vi "Close.vi"(8 "error in (no error)":errorcluster, 11 "ChromaAcLoad in":refnum<class "ChromaAcLoad.lvclass">) -> (0 "error out":errorcluster, 3 "ChromaAcLoad out":refnum<class "ChromaAcLoad.lvclass">)   [LabVIEW 2018, in "AcPwrPlugins.lvlib" / "ChromaAcLoad.lvclass"]
doc: "This VI closes the reference to the instrument(s)."
uses:
  ChromaAcLoad.lvclass
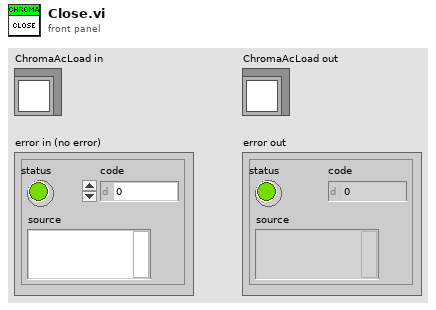
[diagram p1: front panel]
types:
  T1 = typedef "AcPwrPlugins.lvlib/ChromaAcLoad.lvclass/Device(s)Settings.ctl" = cluster{"Configuration Mode":T2, "Phases":cluster{"Handle":string, "Name":string, "Phase Select":i32, "Instrument Options":string, "id query (T)":bool, "reset device (T)":bool, "Load Short Circuited":bool, "Line Synchronization":bool, "Load Current (A/Arms)":dbl, "Load Voltage (V/Vrms)":dbl, "Load Power (W)":dbl, "Load Resistance (Ohms)":dbl, "Load Current Peak Limit (A)":dbl, "Load Current Limit (A/Arms)":dbl, "Load Power Limit (W)":dbl, "Synch Frequency (Hz)":dbl, "Priority":enum16{"CF Only", "PF Only", "Both (CF)", "Both (PF)"}, "Crest Factor":dbl, "Power Factor":dbl, "Slew Rate":cluster{"Rise Slew Rate (A/ms)":i32, "Fall Slew Rate (A/ms)":i32}, "LC/RLC Mode":cluster{"Capacitance (uF)":i32, "Inductance (uH)":i32, "Series Resistance (Ohm)":dbl, "Parallel Resistance (Ohm)":dbl}, "Timing":cluster{"TimingOn":enum16{""}, "Hours":u32, "Minutes":u32, "Seconds":dbl, "CutoffVoltage":dbl}, "Connected":bool}[], "MeasName":string}
  T2 = typedef "ConfigMode.ctl" = enum16{"Constant Voltage (DC)", "Constant Power (DC)", "Constant Power (AC)", "Constant Current (DC)", "Constant Current (AC)", "Constant Resistance (DC)", "Constant Resistance (AC)", "Rectified Mode (DC)", "Inrush (AC)", "RLC CP (AC)", "RLC (AC)"}
  T3 = typedef "AcPwrPlugins.lvlib/ChromaAcLoad.lvclass/Measurements.ctl" = cluster{"Handle":string, "Name":string, "Enabled":bool, "Measurement Value":dbl, "Hold Peak Current Measurement":bool, "btnMeasFetch":bool, "ProtectionStatusString":string, "Measurement Type":T4}[]
  T4 = typedef "AcPwrPlugins.lvlib/ChromaAcLoad.lvclass/MeasurementType.ctl" = enum16{"Voltage (Vrms or V)", "Current (Arms or A)", "Power (W)", "Peak Voltage (V)", "Peak Current (A)", "Peak Power (W)", "Frequency (Hz)", "Resistance (Ohms)", "Voltage Overshoot (V)", "Positive Peak Current (A)", "Voltage Undershoot (V)", "Negative Peak Current (A)", "Apparent Power (VA)", "Reacitive Power (VAR)", "Voltage THD", "Power Factor", "Current's Crest Factor"}
  T5 = cluster{"Handle":string, "Name":string, "Phase Select":i32, "Instrument Options":string, "id query (T)":bool, "reset device (T)":bool, "Load Short Circuited":bool, "Line Synchronization":bool, "Load Current (A/Arms)":dbl, "Load Voltage (V/Vrms)":dbl, "Load Power (W)":dbl, "Load Resistance (Ohms)":dbl, "Load Current Peak Limit (A)":dbl, "Load Current Limit (A/Arms)":dbl, "Load Power Limit (W)":dbl, "Synch Frequency (Hz)":dbl, "Priority":enum16{"CF Only", "PF Only", "Both (CF)", "Both (PF)"}, "Crest Factor":dbl, "Power Factor":dbl, "Slew Rate":cluster{"Rise Slew Rate (A/ms)":i32, "Fall Slew Rate (A/ms)":i32}, "LC/RLC Mode":cluster{"Capacitance (uF)":i32, "Inductance (uH)":i32, "Series Resistance (Ohm)":dbl, "Parallel Resistance (Ohm)":dbl}, "Timing":cluster{"TimingOn":enum16{""}, "Hours":u32, "Minutes":u32, "Seconds":dbl, "CutoffVoltage":dbl}, "Connected":bool}[]
  T6 = cluster{"Handle":string, "Name":string, "Phase Select":i32, "Instrument Options":string, "id query (T)":bool, "reset device (T)":bool, "Load Short Circuited":bool, "Line Synchronization":bool, "Load Current (A/Arms)":dbl, "Load Voltage (V/Vrms)":dbl, "Load Power (W)":dbl, "Load Resistance (Ohms)":dbl, "Load Current Peak Limit (A)":dbl, "Load Current Limit (A/Arms)":dbl, "Load Power Limit (W)":dbl, "Synch Frequency (Hz)":dbl, "Priority":enum16{"CF Only", "PF Only", "Both (CF)", "Both (PF)"}, "Crest Factor":dbl, "Power Factor":dbl, "Slew Rate":cluster{"Rise Slew Rate (A/ms)":i32, "Fall Slew Rate (A/ms)":i32}, "LC/RLC Mode":cluster{"Capacitance (uF)":i32, "Inductance (uH)":i32, "Series Resistance (Ohm)":dbl, "Parallel Resistance (Ohm)":dbl}, "Timing":cluster{"TimingOn":enum16{""}, "Hours":u32, "Minutes":u32, "Seconds":dbl, "CutoffVoltage":dbl}, "Connected":bool}
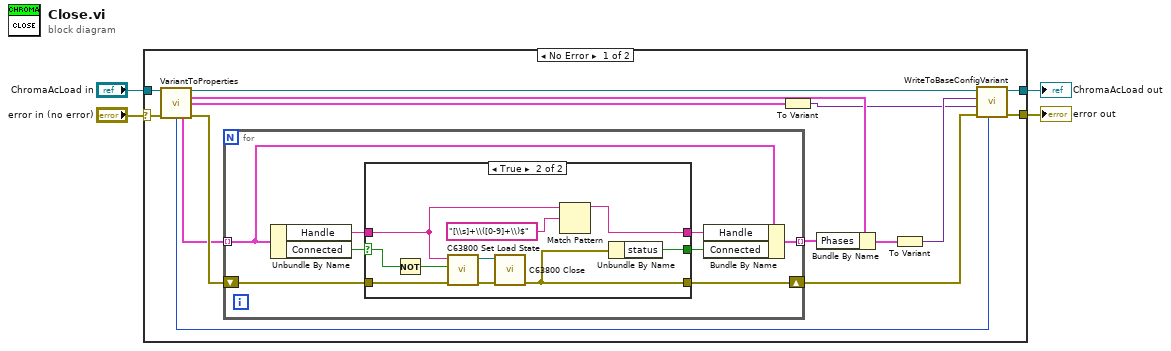
[diagram p0: block diagram]
diagram:
  n1 = case shown="No Error" "error in (no error)" {
    selector: "error in (no error)" -> [w18 w41]
    tunnel: [w9 w42] -> w4
    tunnel: "ChromaAcLoad in" -> [w19 w42]
    tunnel: [w12 w41] -> w1
    frame No Error {
      n2 = call "VariantToProperties.vi"("ChromaAcLoad"=w19, "error in (no error)"=w18) -> ("ChromaAcLoad"=w10:refnum<class "ChromaAcLoad.lvclass">, "Device Properties"=w14:T1, "Meas"=w7:T3, "Measurement Refresh Time (ms)"=w5:u32, "Phases"=w8:T5, "error out"=w16:errorcluster)  [unwired: 7 in, 1 out]
      n3 = for {
        tunnel: w8 -> [w27] mode=indexing
        shift-right: [w25] -> w13
        shift-left: w16 -> [w26]
        tunnel: [w24] -> w17 mode=indexing
        n4 = Unbundle By Name(w27) -> ("Handle"=w23:string, "Connected"=w20:bool)
        n5 = case shown="True" w20 {
          selector: w20 -> [w28 w33]
          tunnel: w23 -> [w29 w32]
          tunnel: w26 -> [w30 w36]
          tunnel: [w30 w38] -> w25
          tunnel: [w29 w39] -> w22
          tunnel: [w28 w37] -> w21
          frame False {
          }
          frame True {
            n6 = Not(x=w33) -> (.not. x?=w34:bool)
            n7 = call <instrlib>:"C63800 Set Load State.vi"("error in (no error)"=w36, "Load State"=w34, "Instrument Handle"=w32) -> ("error out"=w35:errorcluster, "Instrument Handle out"=w31:refnum<k15>)  [unwired: 7 in]
            n8 = call <instrlib>:"C63800 Close.vi"("error in (no error)"=w35, "Instrument Handle"=w31) -> ("error out"=w38:errorcluster)  [unwired: 9 in]
            n9 = Match Pattern(string=w32, regular expression="[\\s]+\\([0-9]+\\)$") -> (before substring=w39:string)  [unwired: 1 in, 3 out]
            n10 = Unbundle By Name(w38) -> ("status"=w37:bool)
          }
        }
        n11 = Bundle By Name(cluster=w27, "Handle"=w22, "Connected"=w21) -> (w24:T6)
      }
      n12 = To Variant(anything=w7) -> (Variant=w6:variant)
      n13 = Bundle By Name(cluster=w14, "Phases"=w17) -> (w15:T1)
      n14 = To Variant(anything=w15) -> (Variant=w11:variant)
      n15 = call-dynamic "WriteToBaseConfigVariant.vi"("Measurement Refresh Time (ms)"=w5, "error in (no error)"=w13, "Meas"=w6, "Config"=w11, "ChromaAcLoad in"=w10) -> ("error out"=w12:errorcluster, "ChromaAcLoad out"=w9:refnum<class "ChromaAcLoad.lvclass">)  [unwired: 5 in]
    }
    frame Error {
    }
  }
  "error out" <- w1
  "ChromaAcLoad out" <- w4
